vi "emi_Error State Changed w init.vi"(9 "Error Inn":errorcluster, 13 "Init(no error)":errorcluster) -> (3 "Changed and Is Error Or Warning":bool, 6 "changed and Is Error":bool, 8 "changed":bool, 10 "error out":errorcluster)   [LabVIEW 2010]
doc: "Monitors a bool, indicateing change, and wheter it was rising or falling. \n\nFirst call will always give out false on all outputs, asuming the previous is the same as the first.\n\nreentrant Subroutine."
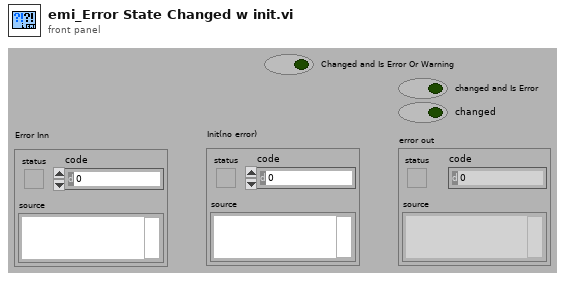
[diagram p1: front panel]
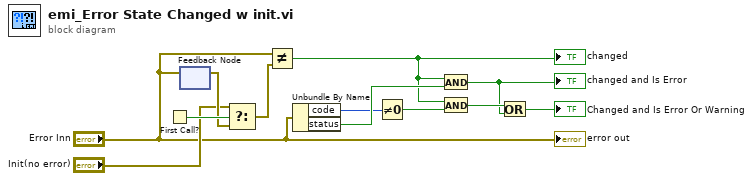
[diagram p0: block diagram]
diagram:
  n1 = First Call?() -> (First Call?: T/F=w12:bool)
  n2 = feedback-in #1("Error Inn") -> ()
  n3 = feedback #1() -> (w11:errorcluster)  [unwired: 1 in]
  n4 = Select(t="Init(no error)", s=w12, f=w11) -> (s? t:f=w10:errorcluster)
  n5 = Not Equal?(x="Error Inn", y=w10) -> (x != y?=w4:bool)
  "changed" <- w4
  n6 = Unbundle By Name("Error Inn") -> ("code"=w6:i32, "status"=w8:bool)
  n7 = Not Equal To 0?(x=w6) -> (x != 0?=w5:bool)
  n8 = And(x=w4, y=w8) -> (x .and. y?=w2:bool)
  "changed and Is Error" <- w2
  n9 = And(x=w4, y=w5) -> (x .and. y?=w3:bool)
  n10 = Or(x=w3, y=w2) -> (x .or. y?=→"Changed and Is Error Or Warning":bool)
  "error out" <- "Error Inn"
